vi "Receive.vi"(10 "Msg in":refnum<class "Msg.lvclass">, 11 "Nominal State in":refnum<class "Nominal State.lvclass">) -> (2 "Msg out":refnum<class "Msg.lvclass">)   [LabVIEW 2021, in "jettl.lvlib" / "Nominal State.lvclass"]
uses:
  Nominal State.lvclass
  Actor/Msg/Msg.lvclass
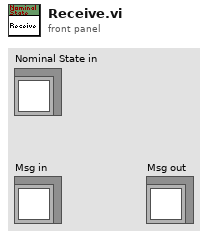
[diagram p1: front panel]
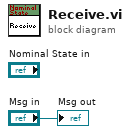
[diagram p0: block diagram]
diagram:
  "Msg out" <- "Msg in"
